vi "ZUP Config Voltage Upper Limit.vi"(8 "error in (no error)":errorcluster, 10 "Voltage Limit":dbl, 11 "VISA resource name":refnum<visa-resource-name>) -> (0 "error out":errorcluster, 2 "Received Message":string, 3 "VISA OUT":refnum<visa-resource-name>)   [LabVIEW 2018]
doc: "Requests the ZUP power supply to set the output voltage to a value specified by the user"
panel:
  # "Lambda TDK ZUP 20-40\nSets the over-voltage limit\nValid Range:\n[01.0 - 24.0]"
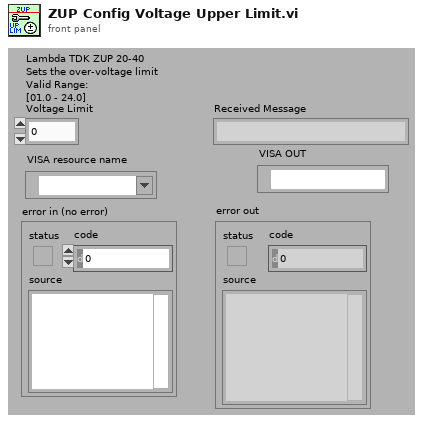
[diagram p1: front panel]
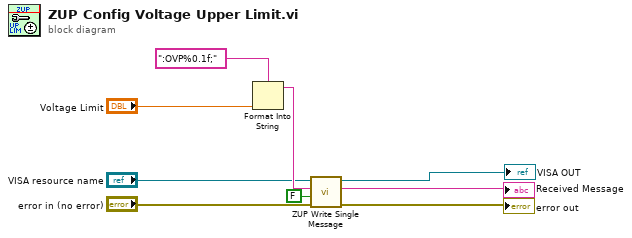
[diagram p0: block diagram]
diagram:
  n1 = Format Into String(format string=":OVP%0.1f;" ("Command Out"), "Voltage Limit") -> (resulting string=w4:string)  [unwired: 2 in, 1 out]
  n2 = call "ZUP Write Single Message.vi"("error in (no error)"="error in (no error)", "Read Response"=FALSE, "Command Out"=w4, "VISA resource name"="VISA resource name") -> ("error out"=→"error out":errorcluster, "Received Message"=→"Received Message":string, "VISA OUT"=→"VISA OUT":refnum<visa-resource-name>)  [unwired: 4 in, 1 out]
